vi "DSF.Execution.Builder.Shutdown.vi"(8 "error in (no error)":errorcluster, 11 "Builder in":refnum<class "DSF.Execution.Builder.lvclass">) -> (0 "error out":errorcluster, 2 "stop?":bool, 3 "Builder out":refnum<class "DSF.Execution.Builder.lvclass">)   [LabVIEW 2016, in "DSF.Execution.lvlib" / "DSF.Execution.Builder.lvclass"]
uses:
  DSF.Execution.Builder.lvclass
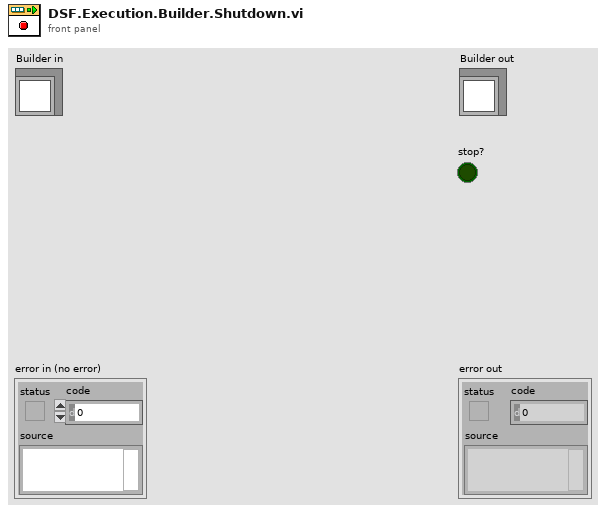
[diagram p1: front panel]
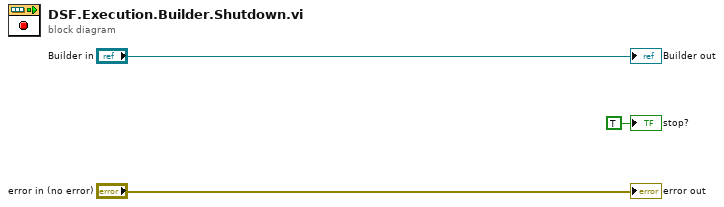
[diagram p0: block diagram]
diagram:
  "error out" <- "error in (no error)"
  "Builder out" <- "Builder in"
  "stop?" <- TRUE ("stop?")
